vi "String to JSON element.vi"(10 "value":string, 11 "keyword":string) -> (2 "JSON last element":string, 3 "JSON element":string)   [LabVIEW 2018]
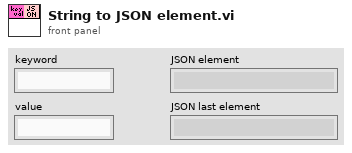
[diagram p1: front panel]
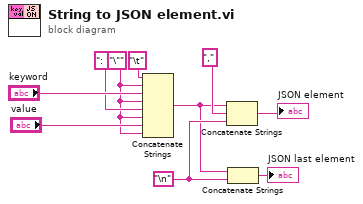
[diagram p0: block diagram]
diagram:
  w4 = "\n"
  w7 = "\""
  n1 = Concatenate Strings("\t", w7, "keyword", w7, ": ", w7, "value", w7) -> (w3:string)
  n2 = Concatenate Strings(w3, ",", w4) -> (→"JSON element":string)
  n3 = Concatenate Strings(w3, w4) -> (→"JSON last element":string)
